vi "Circle detection_new.vi"() -> ()   [LabVIEW 2014]
uses:
  <vilib>/vision/Shape Detection.llb/ShapeDetectionMatchOptions.ctl
  <vilib>/vision/Pattern Matching.llb/IMAQ Match Range Setting.ctl
  <vilib>/vision/Pattern Matching.llb/IMAQ Curve Parameters.ctl
  Resources/Global.vi
  <vilib>/vision/NI_Vision_Development_Module.lvlib
panel:
  out "Radius out":cluster{dbl, dbl}(knob)={0.0, 38.0}
  in  "Target radius":dbl=45.0
  in  "Circle Index":i32
  out "Score":dbl
  out "Number of Matches Returned":i32
  in  "Curve Parameters":T1={"Extraction Mode"=0, "Edge Threshold"=150, "Edge Filter Size"=1, "Min Length"=25, "Row Search Step Size"=15, "Col Search Step Size"=15, "Max Endpoint Gap"=10, "Closed"=TRUE, "Subpixel"=FALSE} {"Extraction Mode" items=["Normal", "Uniform Regions"]; "Edge Filter Size" items=["Fine", "Normal", "Contour Tracing"]; "Max Endpoint Gap" min=0; "Col Search Step Size" min=1 max=255 step=1; "Row Search Step Size" min=1 max=255 step=1; "Min Length" min=0; "Edge Threshold" min=1 max=350 step=1}
  out "error out":errorcluster
  in  "Minimum match score":dbl=900.0
  in  "Match Options":T2={"Rotation"=FALSE, "Scale"=FALSE, "Occlusion"=TRUE, "Range Settings"=[{"Match Constraints"=0, "Min"=0.0, "Max"=0.0}, {"Match Constraints"=1, "Min"=0.0, "Max"=0.0}, {"Match Constraints"=2, "Min"=0.0, "Max"=25.0}]} {"Range Settings"."Max" format="%.2f"; "Range Settings"."Min" format="%.2f"; "Range Settings"."Match Constraints" items=["Rotation Angle (degrees)", "Scale Factor (%)", "Occlusion (%)"]}
  in  "Circle Descriptor":cluster{"Min Radius":dbl, "Max Radius":dbl}={"Min Radius"=20.0, "Max Radius"=400.0}
  out "Image":T4(plugin-control)
  in  "milliseconds to wait":u32
  out "Read Video":errorcluster
  out "x-y":u32=45
  # "Range"
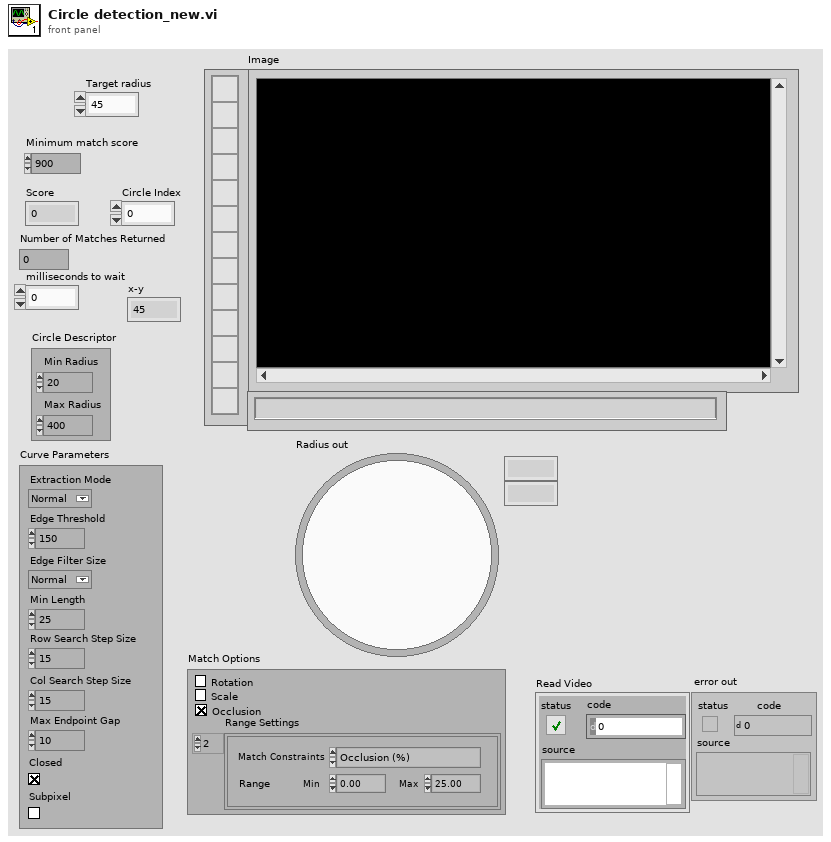
[diagram p1: front panel]
types:
  T1 = typedef "IMAQ Curve Parameters.ctl" = cluster{"Extraction Mode":u32, "Edge Threshold":i32, "Edge Filter Size":u32, "Min Length":i32, "Row Search Step Size":i32, "Col Search Step Size":i32, "Max Endpoint Gap":i32, "Closed":bool, "Subpixel":bool}
  T2 = typedef "ShapeDetectionMatchOptions.ctl" = cluster{"Rotation":bool, "Scale":bool, "Occlusion":bool, "Range Settings":T3[]}
  T3 = typedef "IMAQ Match Range Setting.ctl" = cluster{"Match Constraints":u32, "Min":dbl, "Max":dbl}
  T4 = typedef "IMAQ Image.ctl" = refnum<image>
  T5 = typedef "Image Type" = u32
  T6 = cluster{"Position":cluster{"X":sgl, "Y":sgl}, "Radius":dbl, "Score":dbl}[]
  T7 = cluster{"Position":cluster{"X":sgl, "Y":sgl}, "Radius":dbl, "Score":dbl}
  T8 = cluster{"Left":i32, "Top":i32, "Right":i32, "Bottom":i32}
  T9 = typedef "Control cluster.ctl" = cluster{"Roll":sgl, "Pitch":sgl, "Vertical Speed":sgl, "Yaw Speed":sgl}
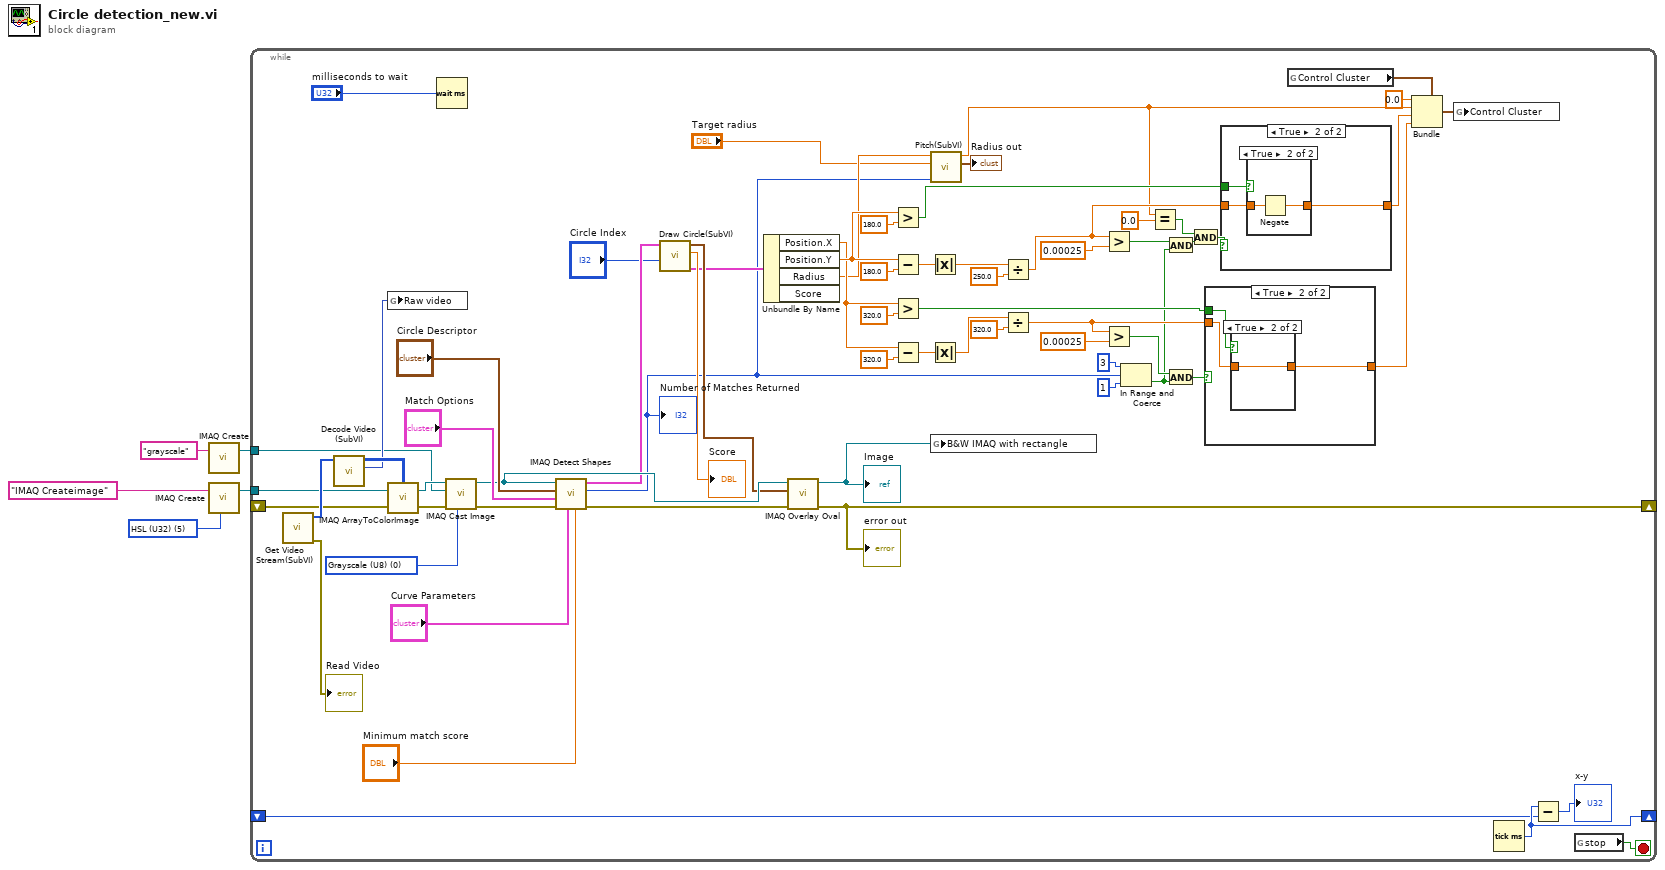
[diagram p0: block diagram]
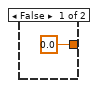
[diagram p2: hidden frame]
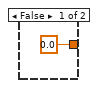
[diagram p4: hidden frame]
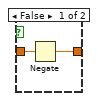
[diagram p5: hidden frame]
diagram:
  w3 = T5 5 items=["Grayscale (U8)", "Grayscale (I16)", "Grayscale (SGL)", "Complex (CSG)", "RGB (U32)", "HSL (U32)", "RGB (U64)", "Grayscale (U16)"] ("Image Type")
  n1 = call "IMAQ Create"("Image Name"="grayscale") -> ("New Image"=w2:T4)  [unwired: 4 in, 1 out]
  n2 = call "IMAQ Create"("Image Name"="IMAQ Createimage", "Image Type"=w3) -> ("New Image"=w4:T4)  [unwired: 3 in, 1 out]
  n3 = while {
    shift-right: [w68] -> _
    shift-left: _ -> [w67]
    shift-right: [w55] -> _
    shift-left: _ -> [w18]
    tunnel: w4 -> [w19]
    tunnel: w2 -> [w17]
    stop <- w26 stop-if-true
    w63 = T5 0 items=["Grayscale (U8)", "Grayscale (I16)", "Grayscale (SGL)", "Complex (CSG)", "RGB (U32)", "HSL (U32)", "RGB (U64)", "Grayscale (U16)"] ("Image Type")
    n4 = call "Get Video Stream(SubVI).vi"() -> ("error out"=→"Read Video":errorcluster, "ImgData"=w71:u8[])  [unwired: 10 in]
    n5 = call "Decode Video (SubVI).vi"("ImgData"=w71) -> ("new picture"=w65:picture, "Array"=w69:u32[][])  [unwired: 9 in]
    n6 = global write "Global.vi" "Raw video"(w65) -> ()
    n7 = call "IMAQ ArrayToColorImage"("Image Pixels (U32)"=w69, "Image"=w19, "error in (no error)"=w18) -> ("Image Out"=w64:T4, "error out"=w20:errorcluster)  [unwired: 2 in]
    n8 = Wait (ms)(milliseconds to wait="milliseconds to wait") -> ()  [unwired: 1 out]
    n9 = call "IMAQ Cast Image"("Image Type"=w63, "error in (no error)"=w20, "Image Dst"=w17, "Image Src"=w64) -> ("error out"=w60:errorcluster, "Image Dst Out"=w58:T4)  [unwired: 6 in]
    n10 = call-poly "IMAQ Detect Shapes"("Minimum match score"="Minimum match score", "Curve Parameters"="Curve Parameters", "error in (no error)"=w60, "Match Options"="Match Options", "Circle Descriptor"="Circle Descriptor", "Image"=w58) -> ("error out"=w57:errorcluster, "Number of Matches Returned"=w14:i32, "Circles"=w53:T6)  [unwired: 3 in]
    "Number of Matches Returned" <- w14
    n11 = call "Draw Circle(SubVI).vi"("Circle Index"="Circle Index", "Circles"=w53) -> ("element"=w51:T7, "Score"=→"Score":dbl, "Bounding Rectangle out"=w56:T8)  [unwired: 7 in]
    n12 = Unbundle By Name(w51) -> ("Position.X"=w36:sgl, "Position.Y"=w41:sgl, "Radius"=w16:dbl)  [unwired: 1 out]
    n13 = call "IMAQ Overlay Oval"("error in (no error)"=w57, "Bounding Rectangle"=w56, "Image"=w58) -> ("error out"=w55:errorcluster, "Image Out"=w49:T4)  [unwired: 7 in]
    "Image" <- w49
    "error out" <- w55
    n14 = Greater?(x=w41, y=180.0) -> (0:w47:bool)
    n15 = Subtract(x=w41, y=180.0) -> (x-y=w44:dbl)
    n16 = Greater?(x=w36, y=320.0) -> (0:w35:bool)
    n17 = Subtract(x=w36, y=320.0) -> (x-y=w39:dbl)
    n18 = Absolute Value(x=w44) -> (abs(x)=w43:dbl)
    n19 = Absolute Value(x=w39) -> (abs(x)=w38:dbl)
    n20 = call <vilib>:"Pitch(SubVI).vi"("Numeric"=w14, "Target radius"="Target radius", "Radius in"=w16) -> ("Radius out"=→"Radius out":cluster{dbl, dbl}, "Pitch out"=w10:sgl)  [unwired: 7 in]
    n21 = global write "Global.vi" "B&W IMAQ with rectangle"(w49) -> ()
    n22 = Divide(x=w43, y=250.0) -> (x/y=w23:dbl)
    n23 = Divide(x=w38, y=320.0) -> (x/y=w33:dbl)
    n24 = Greater?(x=w23, y=0.00025) -> (0:w21:bool)
    n25 = Greater?(x=w33, y=0.00025) -> (0:w30:bool)
    n26 = In Range and Coerce(upper limit=3, x=w14, lower limit=1) -> (In Range?=w24:bool)  [unwired: 1 out]
    n27 = Equal?(x=w10, y=sgl 0.0) -> (x = y?=w11:bool)
    n28 = And(x=w21, y=w24) -> (x .and. y?=w12:bool)
    n29 = And(x=w30, y=w24) -> (x .and. y?=w31:bool)
    n30 = And(x=w11, y=w12) -> (x .and. y?=w13:bool)
    n31 = case shown="True" w31 {
      tunnel: w35 -> [_ w83]
      tunnel: [0.0 w82] -> w34
      tunnel: w33 -> [_ w81]
      frame False {
      }
      frame True {
        n32 = case shown="True" w83 {
          tunnel: w81 -> [w85 w86]
          tunnel: [w84 w86] -> w82
          frame False {
            n33 = Negate(x=w85) -> (-x=w84:dbl)
          }
          frame True {
          }
        }
      }
    }
    n34 = case shown="True" w13 {
      tunnel: w47 -> [_ w76]
      tunnel: w23 -> [_ w75]
      tunnel: [0.0 w74] -> w8
      frame False {
      }
      frame True {
        n35 = case shown="True" w76 {
          tunnel: w75 -> [w77 w79]
          tunnel: [w77 w78] -> w74
          frame False {
          }
          frame True {
            n36 = Negate(x=w79) -> (-x=w78:dbl)
          }
        }
      }
    }
    n37 = global read "Global.vi" "Control Cluster"() -> (w25:T9)
    n38 = Bundle(cluster=w25, "Roll"=sgl 0.0, "Pitch"=w10, "Vertical Speed"=w8, "Yaw Speed"=w34) -> (w50:T9)
    n39 = global write "Global.vi" "Control Cluster"(w50) -> ()
    n40 = Tick Count (ms)() -> (millisecond timer value=w68:u32)
    n41 = Subtract(x=w68, y=w67) -> (x-y=→"x-y":u32)
    n42 = global read "Global.vi" "stop"() -> (w26:bool)
  }
